vi "PCP connected and PC controlled.vi"(1 "Action(GET)":enum16{"GET", "SET"}(ring), 7 "PCP connected  in":bool, 9 "PCP PC controlled in":bool, 11 "error in (no error)":errorcluster) -> (8 "PCP connected out":bool, 10 "PCP PC controlled out":bool, 15 "error out":errorcluster)   [LabVIEW 2011]
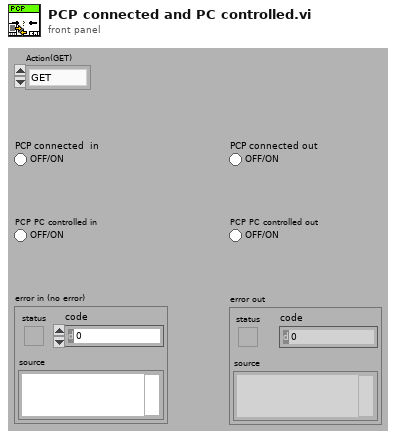
[diagram p1: front panel]
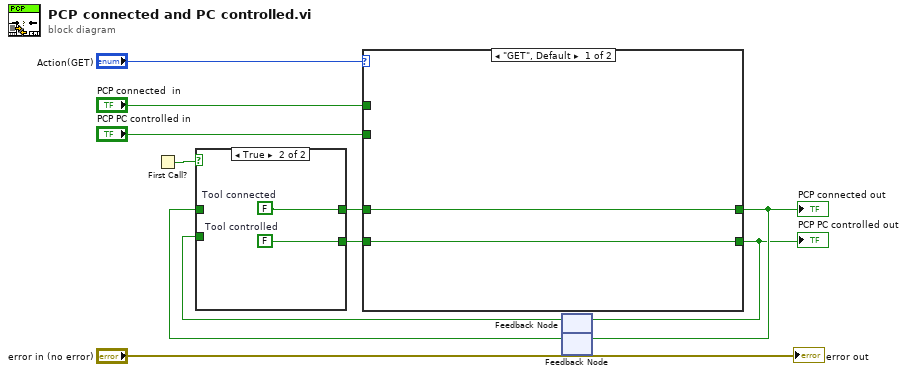
[diagram p0: block diagram]
diagram:
  n1 = First Call?() -> (First Call?: T/F=w8:bool)
  n2 = feedback #1() -> (w2:bool)  [unwired: 1 in]
  n3 = feedback #2() -> (w9:bool)  [unwired: 1 in]
  n4 = case shown="True" w8 {
    tunnel: w9 -> [w13 _]
    tunnel: [w13 w15] -> w6
    tunnel: [w12 w14] -> w3
    tunnel: w2 -> [w12 _]
    frame False {
    }
    frame True {
      w14 = FALSE  # Tool controlled
      w15 = FALSE  # Tool connected
    }
  }
  n5 = case shown="\"GET\", Default" "Action(GET)" {
    tunnel: [w17 w19] -> w7
    tunnel: w6 -> [w17 _]
    tunnel: "PCP connected  in" -> [_ w19]
    tunnel: "PCP PC controlled in" -> [_ w18]
    tunnel: w3 -> [w16 _]
    tunnel: [w16 w18] -> w1
    frame "GET", Default {
    }
    frame "SET" {
    }
  }
  "PCP connected out" <- w7
  "PCP PC controlled out" <- w1
  n6 = feedback-in #1(w1) -> ()
  n7 = feedback-in #2(w7) -> ()
  "error out" <- "error in (no error)"
